vi "FAS.vi"(0 "System no.":i32=1 min=1 step=1, 1 "Board":i32=1 min=1 max=5 step=1, 2 "Axis1 to scan":string, 3 "Axis2 to scan":string, 4 "Area size, deg":dbl=0.2 format="%.4f", 5 "error in":errorcluster, 6 "Treshold level":dbl=0.1 format="%.3f", 7 "Distance between\nscan lines, deg":dbl=0.02 format="%.4f", 10 "Use #7 polling?":bool, 11 "Timeout (s)":dbl=300.0 min=1.0 max=4.0 step=1.0 format="%.2f", 12 "Stop refnum":refnum<vi>) -> (14 "Scan successful?":bool, 19 "error out":errorcluster)   [LabVIEW 2020]
doc: "Performs a fast angular scan in specified axes, waits until scan is finished (using #7 polling if checked) and indicates whether scan was successful or not. \"Timeout\" is only valid if \"Use #7 polling\" is FALSE. If Refnum stop or Local stop is TRUE, VI sends #24 and stops. \n\nC-887, F-206: Use #7 polling = FALSE. Only for GCS syntax version = GCS 1.0 (check with CSV?.vi. If CSV?.vi is not supported, syntax version is GCS 1.0). For compatibility reasons, VI calls FSC automatically for GCS 2.0."
uses:
  Communication.llb/Syntax.ctl
  Communication.llb/Global1.vi
panel:
  in  "Local stop":bool
  # "Performs a fast angular scan in specified axes, waits until scan is finished (using #7 polling if checked) and \nindicates whether scan was successful or not. \"Timeout\" is only valid if \"Use #7 polling\" is FALSE. If Stop refnum or Local \nstop is TRUE, VI sends #24 and stops."
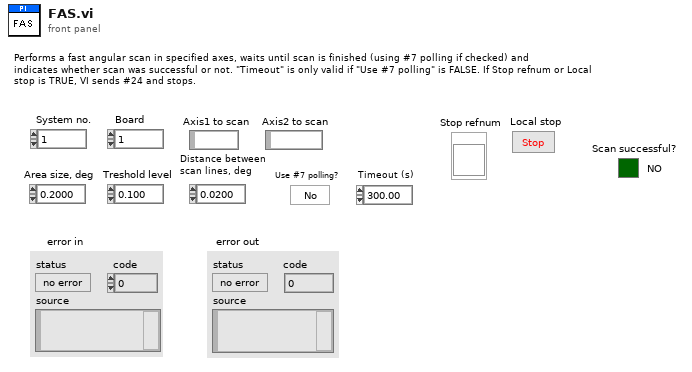
[diagram p1: front panel]
types:
  T1 = typedef "Syntax.ctl" = enum16{"GCS 1.0", "GCS 2.0", "GCS 3.0"}
  T2 = enum16{"Disable error check", "Force error check", "Use global settings"}
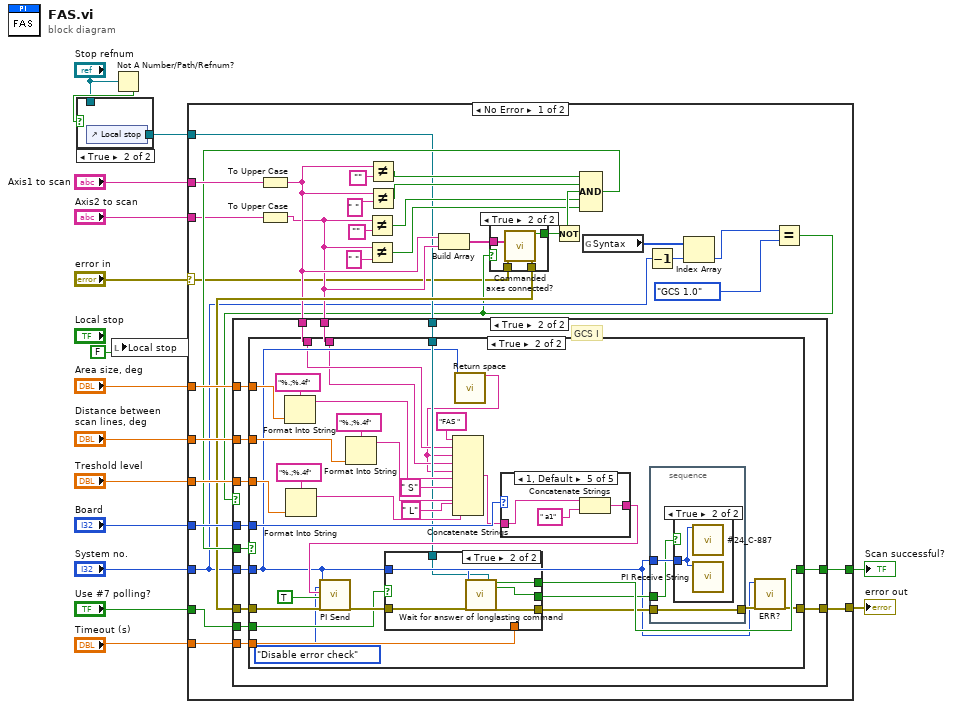
[diagram p0: block diagram]
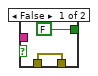
[diagram p3: hidden frame]
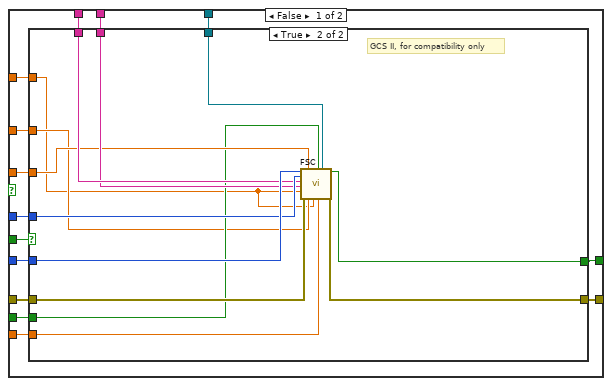
[diagram p4: hidden frame]
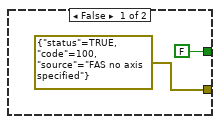
[diagram p5: hidden frame]
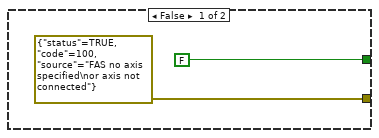
[diagram p6: hidden frame]
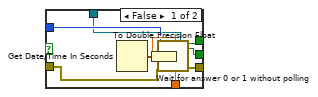
[diagram p7: hidden frame]
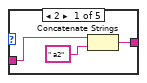
[diagram p9: hidden frame]
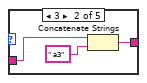
[diagram p10: hidden frame]
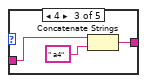
[diagram p11: hidden frame]
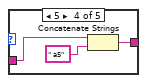
[diagram p12: hidden frame]
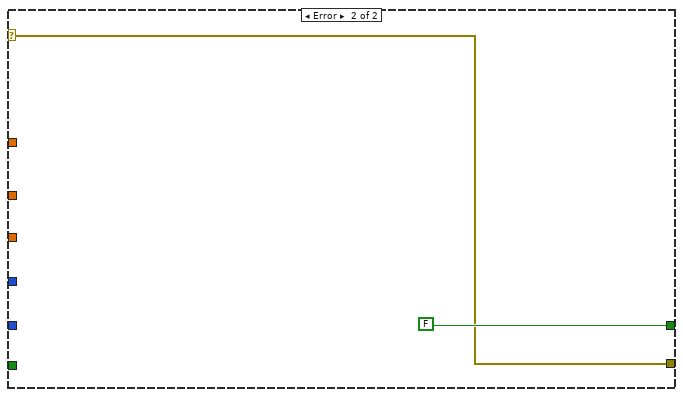
[diagram p13: hidden frame]
diagram:
  n1 = local write "Local stop"(FALSE ("Local stop")) -> ()
  n2 = Not A Number/Path/Refnum?(number/path/refnum="Stop refnum") -> (NaN/Path/Refnum?=w4:bool)
  n3 = case shown="True" w4 {
    tunnel: [w17 w18] -> w2
    tunnel: "Stop refnum" -> [w17 _]
    frame False {
    }
    frame True {
      n4 = control-ref of="Local stop"() -> (w18:refnum<vi>)
    }
  }
  n5 = case shown="No Error" "error in" {
    selector: "error in" -> [w20 w168]
    tunnel: "System no." -> [w22 _]
    tunnel: [w39 w168] -> w15
    tunnel: "Axis1 to scan" -> [w51 _]
    tunnel: [w38 FALSE] -> w13
    tunnel: "Board" -> [w45 _]
    tunnel: "Area size, deg" -> [w44 _]
    tunnel: "Distance between\nscan lines, deg" -> [w43 _]
    tunnel: "Treshold level" -> [w42 _]
    tunnel: "Use #7 polling?" -> [w35 _]
    tunnel: "Axis2 to scan" -> [w32 _]
    tunnel: "Timeout (s)" -> [w27 _]
    tunnel: w2 -> [w26 _]
    frame No Error {
      n6 = To Upper Case(1:w51) -> (0:w29:string)
      n7 = To Upper Case(1:w32) -> (0:w28:string)
      n8 = Not Equal?(x=w28, y="") -> (x != y?=w31:bool)
      n9 = Not Equal?(x=w28, y=" ") -> (x != y?=w30:bool)
      n10 = Not Equal?(x=w29, y="") -> (x != y?=w48:bool)
      n11 = Not Equal?(x=w29, y=" ") -> (x != y?=w47:bool)
      n12 = Build Array(w29, w28) -> (w46:string[])
      n13 = global read "Global1.vi" "Syntax"() -> (w23:T1[])
      n14 = Decrement(x=w22) -> (x-1=w24:i32)
      n15 = Index Array(array=w23, index=w24) -> (element=w25:T1)
      n16 = Equal?(x=w25, y=Syntax."GCS 1.0") -> (x = y?=w21:bool)
      n17 = case shown="True" w21 {
        tunnel: w46 -> [_ w57]
        tunnel: w20 -> [w53 w56]
        tunnel: [w53 w55] -> w40
        tunnel: [FALSE ("Controller error") w54] -> w37
        frame False {
        }
        frame True {
          n18 = call "Commanded axes connected?.vi"("Commanded axes"=w57, "error in"=w56) -> ("Controller error"=w54:bool, "error out"=w55:errorcluster)  [unwired: 1 in, 15 out]
        }
      }
      n19 = Not(x=w37) -> (.not. x?=w36:bool)
      n20 = Compound Arithmetic op=AND(w48, w47, w36, w31, w30) -> (w41:bool)
      n21 = case shown="True" w21 {
        tunnel: w45 -> [w67 w100]
        tunnel: w44 -> [w64 w99]
        tunnel: w43 -> [w60 w98]
        tunnel: w42 -> [w62 w97]
        tunnel: w41 -> [w71 w96]
        tunnel: w40 -> [w63 w95]
        tunnel: w22 -> [w68 w94]
        tunnel: [w70 w93] -> w39
        tunnel: [w69 w92] -> w38
        tunnel: w35 -> [w61 w91]
        tunnel: w29 -> [w66 w90]
        tunnel: w28 -> [w65 w89]
        tunnel: w27 -> [w58 w88]
        tunnel: w26 -> [w59 w87]
        frame False {
          n22 = case shown="True" w71 {
            tunnel: [errorcluster {"status"=TRUE, "code"=100, "source"="FAS no axis specified"} ("error out") w74] -> w70
            tunnel: [FALSE w75] -> w69
            tunnel: w68 -> [_ w86]
            tunnel: w67 -> [_ w85]
            tunnel: w66 -> [_ w84]
            tunnel: w65 -> [_ w83]
            tunnel: w64 -> [_ w77]
            tunnel: w63 -> [_ w82]
            tunnel: w62 -> [_ w81]
            tunnel: w61 -> [_ w80]
            tunnel: w60 -> [_ w79]
            tunnel: w59 -> [_ w78]
            tunnel: w58 -> [_ w76]
            frame False {
            }
            frame True {
              # "GCS II, for compatibility only"
              n23 = call "FSC.vi"("System no."=w86, "Board"=w85, "Axis 1 to scan"=w84, "Axis 2 to scan"=w83, "Range axis 1"=w77, "error in"=w82, "Treshold level"=w81, "Step size"=w79, "Range axis 2"=w77, "Use #7 polling?"=w80, "Timeout (s)"=w76, "Stop refnum"=w78) -> ("Scan successful?"=w75:bool, "error out"=w74:errorcluster)  [unwired: 6 out]
            }
          }
        }
        frame True {
          # "GCS I"
          n24 = case shown="True" w96 {
            tunnel: w100 -> [_ w133]
            tunnel: w99 -> [_ w123]
            tunnel: w98 -> [_ w117]
            tunnel: w90 -> [_ w106]
            tunnel: w97 -> [_ w119]
            tunnel: w95 -> [_ w128]
            tunnel: w94 -> [_ w108]
            tunnel: [errorcluster {"status"=TRUE, "code"=100, "source"="FAS no axis specified\nor axis not connected"} ("error out") w113] -> w93
            tunnel: [FALSE w125] -> w92
            tunnel: w91 -> [_ w112]
            tunnel: w89 -> [_ w105]
            tunnel: w88 -> [_ w111]
            tunnel: w87 -> [_ w110]
            frame False {
            }
            frame True {
              n25 = Format Into String(format string="%.;%.4f" ("Format String"), w123) -> (resulting string=w122:string)  [unwired: 2 in, 1 out]
              n26 = Format Into String(format string="%.;%.4f" ("Format String"), w119) -> (resulting string=w120:string)  [unwired: 2 in, 1 out]
              n27 = Format Into String(format string="%.;%.4f" ("Format String"), w117) -> (resulting string=w116:string)  [unwired: 2 in, 1 out]
              n28 = call "Return space.vi"("System no."=w108) -> ("String out"=w104:string)  [unwired: 1 in, 17 out]
              n29 = Concatenate Strings("FAS ", w106, w104, w105, w104, w122, " S", w116, " L", w120) -> (w132:string)
              n30 = case shown="1, Default" w133 {
                tunnel: w132 -> [w155 w158 w161 w164 w167]
                tunnel: [w153 w156 w159 w162 w165] -> w129
                frame 2 {
                  n31 = Concatenate Strings(w155, " a2" ("Substring")) -> (w153:string)
                }
                frame 3 {
                  n32 = Concatenate Strings(w158, " a3" ("Substring")) -> (w156:string)
                }
                frame 4 {
                  n33 = Concatenate Strings(w161, " a4" ("Substring")) -> (w159:string)
                }
                frame 5 {
                  n34 = Concatenate Strings(w164, " a5" ("Substring")) -> (w162:string)
                }
                frame 1, Default {
                  n35 = Concatenate Strings(w167, " a1" ("Substring")) -> (w165:string)
                }
              }
              n36 = call "PI Send.vi"("System no."=w108, "Error check settings"=T2."Disable error check", "String to send"=w129, "Attach termination char.?"=TRUE ("Attach Linefeed?"), "error in"=w128) -> ("error out"=w126:errorcluster)  [unwired: 1 in, 13 out]
              n37 = case shown="True" w112 {
                tunnel: w126 -> [w139 w148]
                tunnel: [w141 w147] -> w125
                tunnel: [w140 w146] -> w115
                tunnel: w108 -> [w137 w145]
                tunnel: w111 -> [w138 _]
                tunnel: w110 -> [w136 w144]
                tunnel: [w135 w143] -> w109
                frame False {
                  n38 = Get Date/Time In Seconds() -> (seconds since 1Jan1904=w134:timestamp)
                  n39 = To Double Precision Float(number=w134) -> (double precision float=w142:dbl)
                  n40 = call "Wait for answer 0 or 1 without polling.vi"("System no."=w137, "error in"=w139, "Start time"=w142, "Timeout (s)"=w138, "Stop refnum"=w136) -> ("Scan successful?"=w141:bool, "Stopped"=w135:bool, "error out"=w140:errorcluster)  [unwired: 12 out]
                }
                frame True {
                  n41 = call "Wait for answer of longlasting command.vi"("System no."=w145, "error in"=w148, "Stop refnum"=w144) -> ("Answer"=w147:bool, "Stopped"=w143:bool, "error out"=w146:errorcluster)  [unwired: 14 out]
                }
              }
              n42 = stacked-sequence {
                tunnel: w108 -> [w151]
                tunnel: [w150] -> w114
                tunnel: w115 -> [w150]
                tunnel: w109 -> [w149]
                frame #0 {
                  n43 = case shown="True" w149 {
                    tunnel: w151 -> [_ w152]
                    frame False {
                    }
                    frame True {
                      n44 = call "#24_C-887.vi"("System no."=w152) -> ()  [unwired: 1 in, 18 out]
                      n45 = call "PI Receive String.vi"("System no."=w152) -> ()  [unwired: 2 in, 17 out]
                    }
                  }
                }
              }
              n46 = call "ERR?.vi"("System no."=w108, "error in"=w114) -> ("error out"=w113:errorcluster)  [unwired: 17 out]
            }
          }
        }
      }
    }
    frame Error {
    }
  }
  "error out" <- w15
  "Scan successful?" <- w13
